vi "ws_get_use.vi"(0 "target_name":string) -> (1 "in_use":bool, 2 "user":string, 3 "Error?":bool, 4 "Error_info":string)   [LabVIEW 2011]
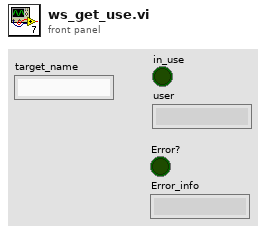
[diagram p1: front panel]
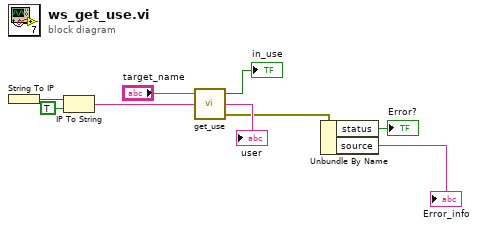
[diagram p0: block diagram]
diagram:
  n1 = String To IP() -> (0:w9:u32)  [unwired: 1 in]
  n2 = IP To String(1:TRUE ("dot notation? (F)"), 2:w9) -> (0:w7:string)
  n3 = call "get_use.vi"("Remote Server Address"=w7, "Target Name"="target_name") -> ("error out"=w3:errorcluster, "user"=→"user":string, "in use?"=→"in_use":bool)  [unwired: 1 in]
  n4 = Unbundle By Name(w3) -> ("status"=→"Error?":bool, "source"=→"Error_info":string)
